vi "need for local.vi"() -> ()   [LabVIEW 2013]
panel:
  in  "stop":bool
  out "Loop 2 executed":bool
  in  "ON/OFF":bool
  out "Loop 1 executed":bool
  in  "ON/OFF":bool
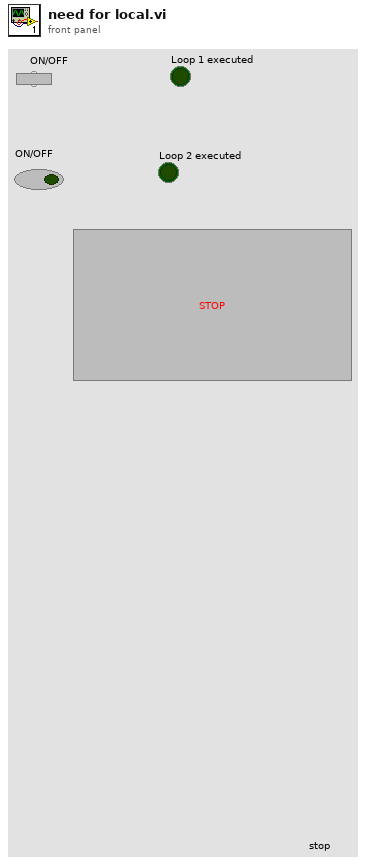
[diagram p1: front panel]
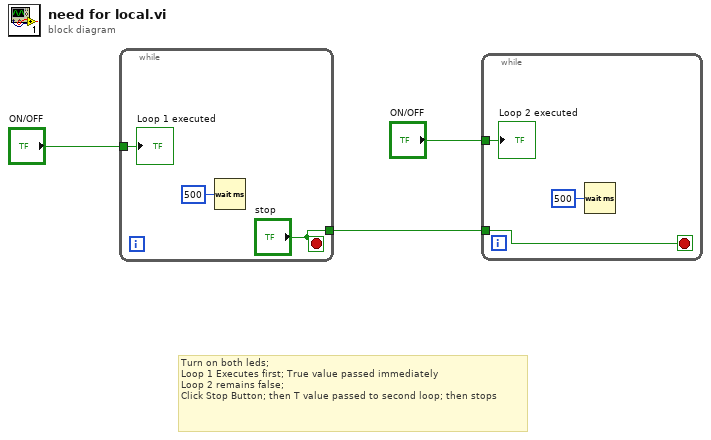
[diagram p0: block diagram]
diagram:
  # "Turn on both leds;\nLoop 1 Executes first; True value passed immediately\nLoop 2 remains false;\nClick Stop Button; then T value passed to second loop; then stops"
  n1 = while {
    tunnel: "ON/OFF" -> [w6]
    tunnel: ["stop"] -> w1
    stop <- "stop" stop-if-true
    n2 = Wait (ms)(milliseconds to wait=u32 500) -> ()  [unwired: 1 out]
    "Loop 1 executed" <- w6
  }
  n3 = while {
    tunnel: "ON/OFF" -> [w9]
    tunnel: w1 -> [w7]
    stop <- w7 stop-if-true
    n4 = Wait (ms)(milliseconds to wait=u32 500) -> ()  [unwired: 1 out]
    "Loop 2 executed" <- w9
  }
